vi "potential_v1.vi"() -> ()   [LabVIEW 2009]
panel:
  in  "sig":ext(slide)=0.010303486529318543 scale=0.01..0.015
  in  "eps":dbl(slide)=10.0 scale=0.0..10.0
  in  "stop":bool
  out "Lennard-Jones potential":cluster{dbl[], dbl[]}(graph)={[0.01, 0.02, 0.03, 0.04, 0.05, 0.060000000000000005, 0.07, 0.08, 0.09, 0.09999999999999999, 0.10999999999999999, 0.11999999999999998, 0.12999999999999998, 0.13999999999999999, 0.15, 0.16, 0.17, 0.18000000000000002, 0.19000000000000003, 0.20000000000000004, 0.21000000000000005, 0.22000000000000006, 0.23000000000000007, 0.24000000000000007, 0.25000000000000006, 0.26000000000000006, 0.2700000000000001, 0.2800000000000001, 0.2900000000000001, 0.3000000000000001, 0.3100000000000001, 0.3200000000000001, 0.3300000000000001, 0.34000000000000014, 0.35000000000000014, 0.36000000000000015, 0.37000000000000016, 0.38000000000000017, 0.3900000000000002, 0.4000000000000002, 0.4100000000000002, 0.4200000000000002, 0.4300000000000002, 0.4400000000000002, 0.45000000000000023, 0.46000000000000024, 0.47000000000000025, 0.48000000000000026, 0.49000000000000027, 0.5000000000000002, 0.5100000000000002, 0.5200000000000002, 0.5300000000000002, 0.5400000000000003, 0.5500000000000003, 0.5600000000000003, 0.5700000000000003, 0.5800000000000003, 0.5900000000000003, 0.6000000000000003, 0.6100000000000003, 0.6200000000000003, 0.6300000000000003, 0.6400000000000003, 0.6500000000000004, 0.6600000000000004, 0.6700000000000004, 0.6800000000000004, 0.6900000000000004, 0.7000000000000004, 0.7100000000000004, 0.7200000000000004, 0.7300000000000004, 0.7400000000000004, 0.7500000000000004, 0.7600000000000005, 0.7700000000000005, 0.7800000000000005, 0.7900000000000005, 0.8000000000000005, 0.8100000000000005, 0.8200000000000005, 0.8300000000000005, 0.8400000000000005, 0.8500000000000005, 0.8600000000000005, 0.8700000000000006, 0.8800000000000006, 0.8900000000000006, 0.9000000000000006, 0.9100000000000006, 0.9200000000000006, 0.9300000000000006, 0.9400000000000006, 0.9500000000000006, 0.9600000000000006, 0.9700000000000006, 0.9800000000000006, 0.9900000000000007, 1.0000000000000007], [1.250787746665296, -9.990789592652218, -9.01967827643145, -7.649440662822326, -6.544199868897255, -5.689415078880709, -5.021079366468974, -4.488231798035217, -4.055071372734915, -3.6967472730880226, -3.3957741605460865, -3.1396015246066016, -2.9190329329031055, -2.72719648866275, -2.5588642573118805, -2.409993765673622, -2.2774129762274096, -2.1585996797746776, -2.0515242170755394, -1.9545354712038596, -1.8662769492036688, -1.785624133710934, -1.7116371017643974, -1.6435242585948617, -1.5806142705086634, -1.522334120096433, -1.4681917850513895, -1.4177624456884401, -1.370677412053521, -1.3266151662825392, -1.2852940642784176, -1.246466349500814, -1.2099132121268206, -1.1754406869579428, -1.1428762287678824, -1.1120658382391435, -1.0828716380388637, -1.0551698189698604, -1.028848891985373, -1.0038081942668917, -0.9799566073434269, -0.9572114529827522, -0.9354975387662785, -0.9147463302149397, -0.8948952303276037, -0.8758869506288618, -0.8576689604562905, -0.8401930033703211, -0.8234146713379816, -0.8072930287999073, -0.7917902799373481, -0.7768714734594365, -0.7625042400682059, -0.7486585584598302, -0.7353065463094673, -0.7224222731834863, -0.7099815927425938, -0.6979619919553988, -0.6863424553447961, -0.6751033425479194, -0.6642262776914226, -0.6536940492734281, -0.6434905194064833, -0.6336005414164078, -0.6240098849133444, -0.6147051675565093, -0.6056737928254463, -0.5969038931900309, -0.5883842781407218, -0.5801043866010717, -0.5720542432974658, -0.5642244187075229, -0.5566059922494039, -0.5491905184102168, -0.5419699955433994, -0.5349368370929528, -0.5280838450271833, -0.5214041852865621, -0.5148913650698155, -0.5085392117996863, -0.5023418536252502, -0.49629370133143075, -0.49038943153865794, -0.48462397108660554, -0.4789924825057942, -0.4734903504896751, -0.46811316928774094, -0.462856730947338, -0.4577170143382729, -0.45269017490009056, -0.4477725350571196, -0.4429605752510966, -0.43825092554544526, -0.43364035775914783, -0.4291257780916459, -0.42470422020338305, -0.42037283871948694, -0.4161289031267104, -0.41196979203613926, -0.40789298778634747]}
  out "r":dbl=1.0000000000000007
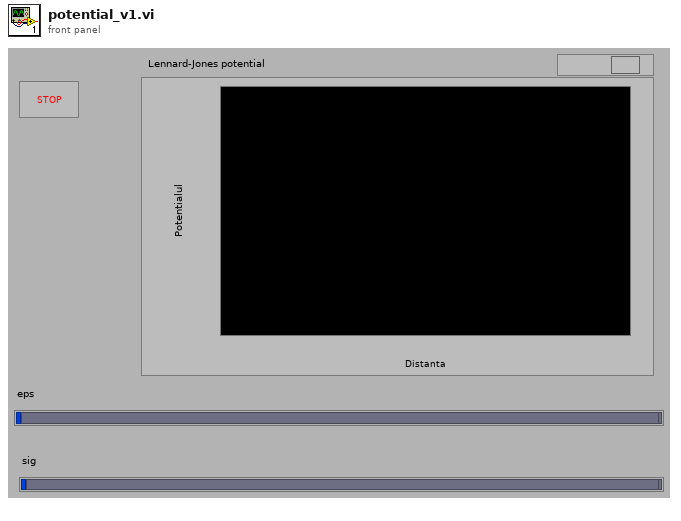
[diagram p1: front panel]
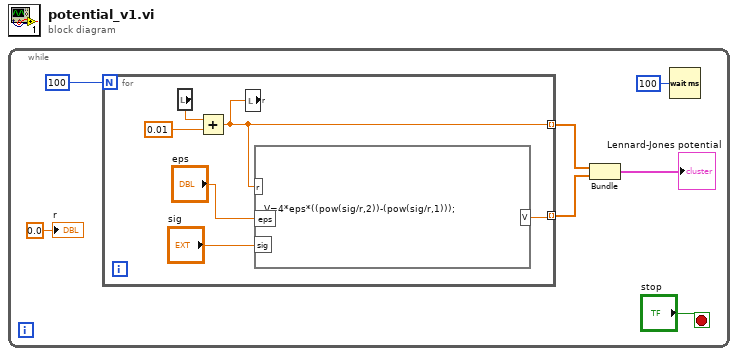
[diagram p0: block diagram]
diagram:
  n1 = while {
    stop <- "stop" stop-if-true
    n2 = for {
      N: 100 -> [_]
      tunnel: [w8] -> w5 mode=indexing
      tunnel: [w12] -> w4 mode=indexing
      n3 = local read "r"() -> (w13:dbl)
      n4 = Add(x=w13, y=0.01) -> (x+y=w8:dbl)
      n5 = local write "r"(w8) -> ()
      n6 = formula code="V=4*eps*((pow(sig/r,2))-(pow(sig/r,1)));"("r"=w8, "eps"="eps", "sig"="sig") -> ("V"=w12:dbl)
    }
    n7 = Bundle(w5, w4) -> (→"Lennard-Jones potential":cluster{dbl[], dbl[]})  [unwired: 1 in]
    n8 = Wait (ms)(milliseconds to wait=u32 100) -> ()  [unwired: 1 out]
    "r" <- 0.0 ("r")
  }
